vi "Main.vi"(11 "Module Admin":refnum<class "Delacor_lib_QMH_Module Admin.lvclass">) -> ()   [LabVIEW 2019, in "Acquisition.lvlib"]
doc: "This template is based off of the Queued Message Handler design pattern and the Queued Message Handler project template that ships with LabVIEW.\n\nThe main difference is that the queue is private to this module and communication between modules is performed via Broadcast and Request events.\n\nRequest events are wrapped in public API methods and are handled in the Event Handling Loop (EHL) of this VI. Any module can register for Broadcast events sent by this module. The EHL generates messages based on user interface actions.\n\nThe Message Handling Loop (MHL) processes messages generated by the EHL, or by other messages. The messages are string values, so new messages can be added easily to the Message Cases case structure in the MHL. Each message cluster can also provide an optional value for Message Data, which is a variant that can be converted to whatever message-specific data is required.\n_____\nBased on Delacor QMH Project Template 5.0.0.82."
uses:
  Acquisition.lvlib
  <vilib>/Delacor/Delacor QMH/Libraries/Module Admin_class/Delacor_lib_QMH_Module Admin.lvclass
  Module Data--cluster.ctl
  <vilib>/Delacor/Delacor QMH/Libraries/Message Queue_class/Delacor_lib_QMH_Message Queue.lvclass/Delacor_lib_QMH_Message Queue.ctl
  Stop Argument--cluster.ctl
  <vilib>/Delacor/Delacor QMH/Libraries/Module Admin_class/Delacor_lib_QMH_Module Admin.lvclass/Delacor_lib_QMH_Module Admin.ctl
  <vilib>/Utility/miscctls.llb/LVPointTypeDef.ctl
  <vilib>/Delacor/Delacor QMH/Libraries/Message Queue_class/Delacor_lib_QMH_Enqueue Message (Single).vi
  <vilib>/Delacor/Delacor QMH/Libraries/Module Admin_class/Delacor_lib_QMH_Get External Launch.vi
  <vilib>/Utility/error.llb/Error Cluster From Error Code.vi
  <vilib>/ErrorRing/Error Ring.xnode
  <vilib>/Delacor/Delacor QMH/Libraries/Message Queue_class/Delacor_lib_QMH_Message Queue.lvclass
panel:
  in  "Simulate MHL Error":bool
  in  "Simulate EHL Error":bool
  out "error out":errorcluster
  out "Status":string
types:
  T1 = typedef "Acquisition.lvlib/Request Events--cluster.ctl" = cluster{"Stop Module":refnum<user-event>, "Show Panel":refnum<user-event>, "Hide Panel":refnum<user-event>, "Get Module Execution Status":refnum<user-event>, "Show Diagram":refnum<user-event>}
  T2 = typedef "Acquisition.lvlib/Module Data--cluster.ctl" = cluster{"Status":string}
  T3 = enum32{"invalid lock state", "Not Locked", "Locked (No Password)", "Password-protected"}
  T4 = typedef "Acquisition.lvlib/Stop Argument--cluster.ctl" = cluster{"Origin":string, "Exit via Stop Module Req?":bool, "Wait for Module to stop?":bool}
  T5 = typedef "LVPointTypeDef.ctl" = cluster{"Horizontal":i16, "Vertical":i16}
  T6 = enum32{"Invalid", "Standard", "Closed", "Hidden", "Minimized", "Maximized"}
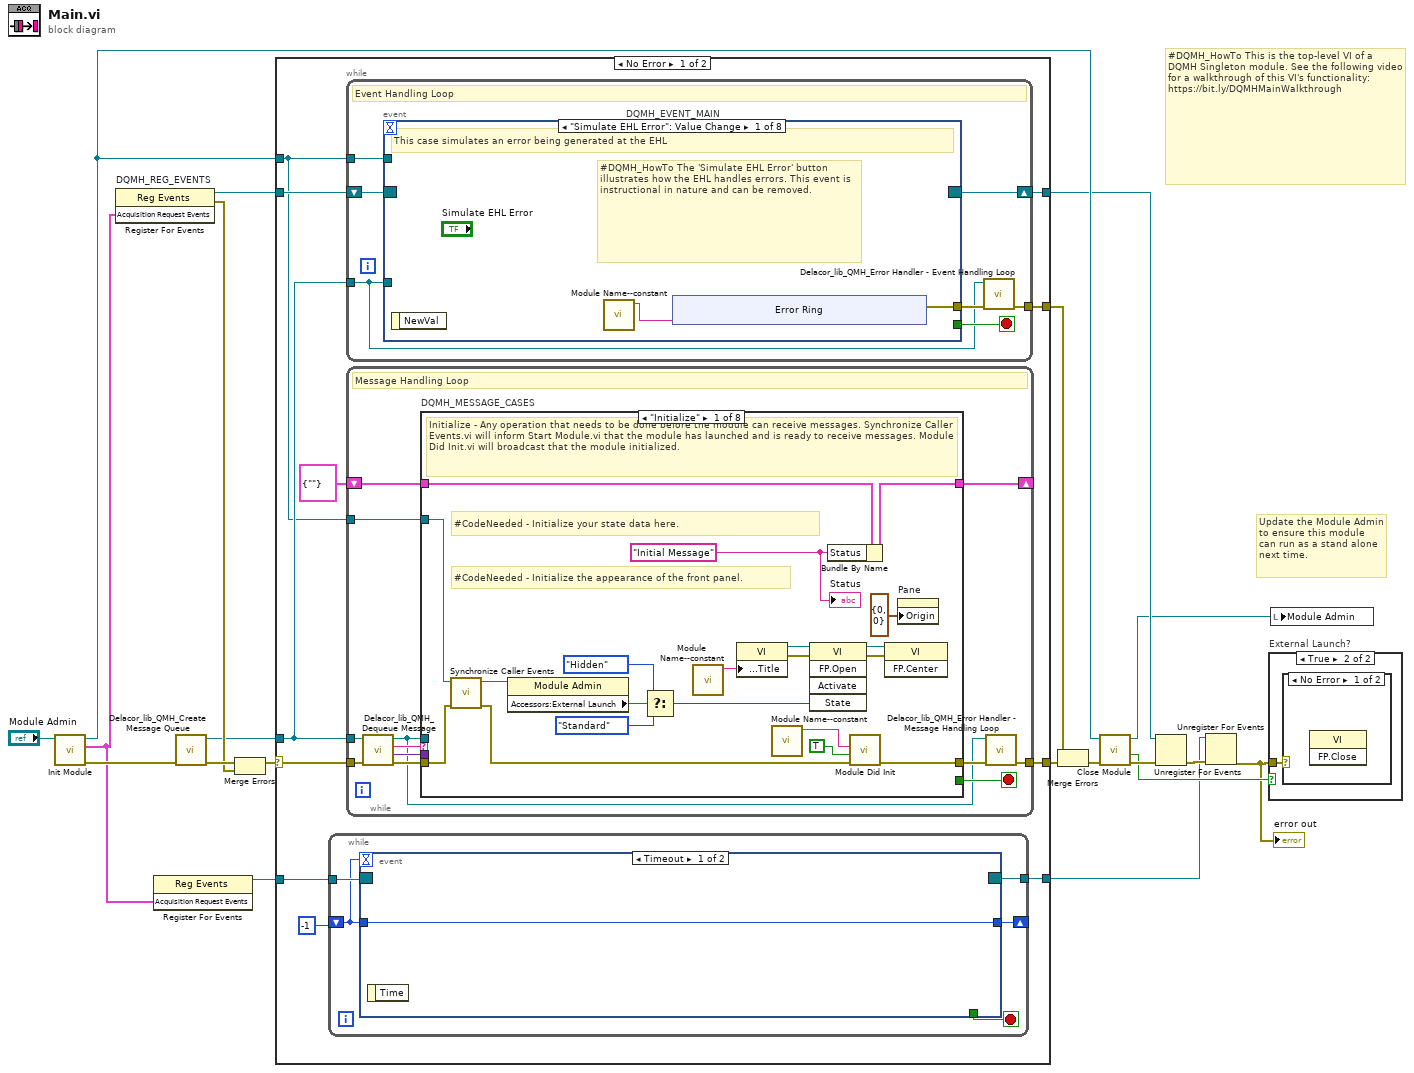
[diagram p0: block diagram]
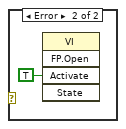
[diagram p3: hidden frame]
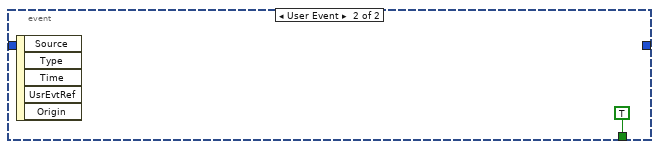
[diagram p4: hidden frame]
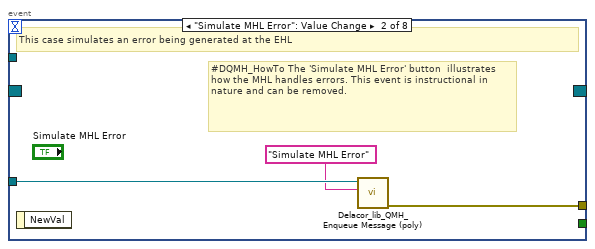
[diagram p5: hidden frame]
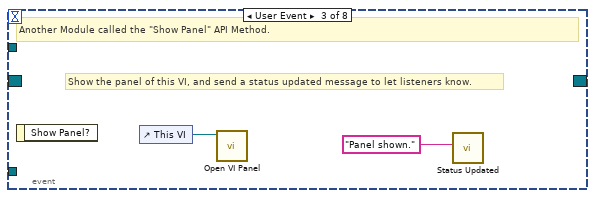
[diagram p6: hidden frame]
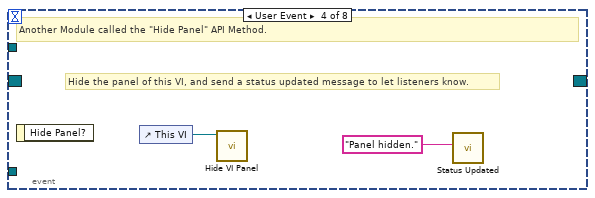
[diagram p7: hidden frame]
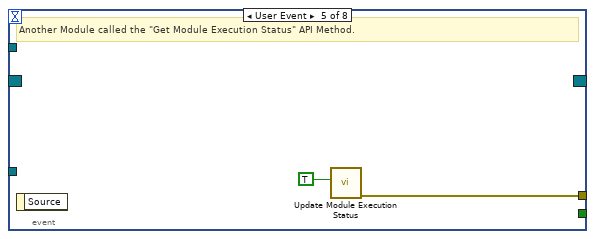
[diagram p8: hidden frame]
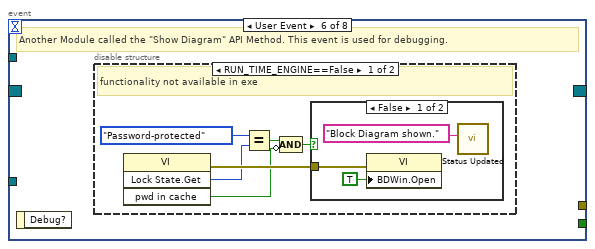
[diagram p9: hidden frame]
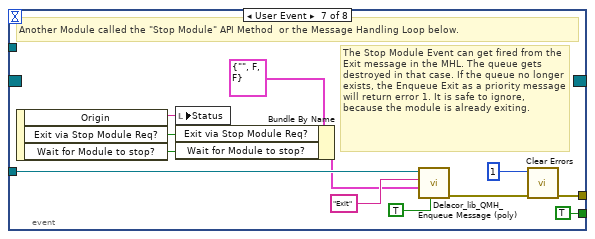
[diagram p12: hidden frame]
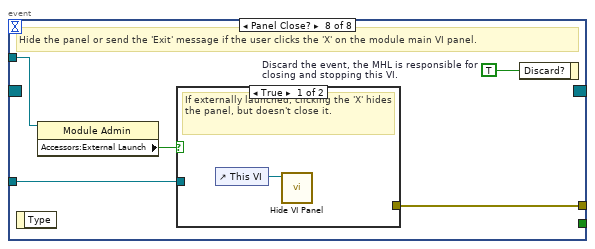
[diagram p13: hidden frame]
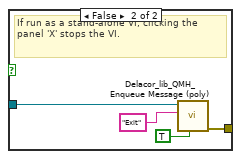
[diagram p14: hidden frame]
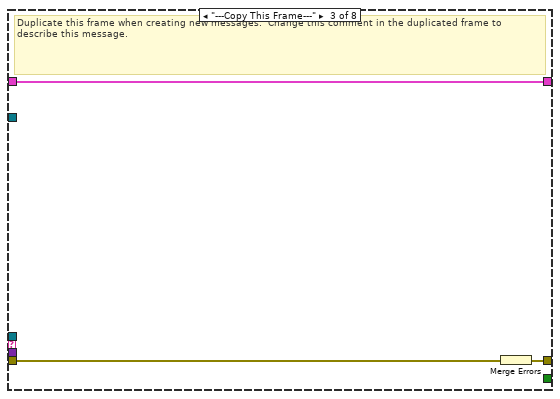
[diagram p16: hidden frame]
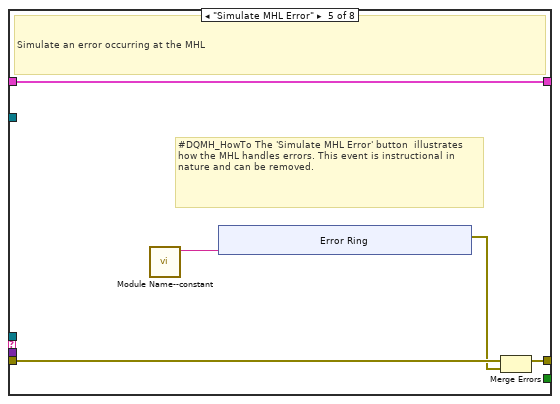
[diagram p18: hidden frame]
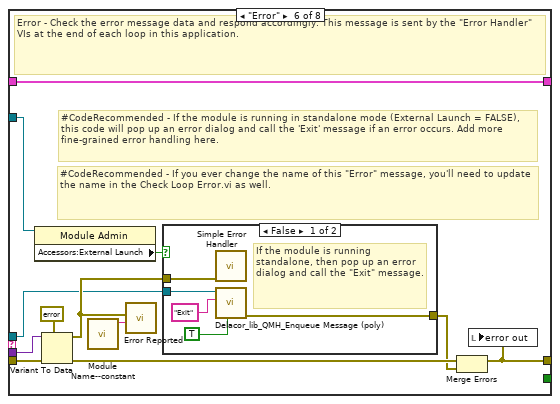
[diagram p19: hidden frame]
diagram:
  # "#DQMH_HowTo This is the top-level VI of a DQMH Singleton module. See the following video for a walkthrough of this VI's functionality: https://bit.ly/DQMHMainWalkthrough"
  # "Update the Module Admin to ensure this module can run as a stand alone next time."
  n1 = call "Init Module.vi"("Singleton Module Admin in"="Module Admin") -> ("error out"=w19:errorcluster, "Acquisition Request Events"=w5:T1, "Singleton Module Admin out"=w12:refnum<class "Delacor_lib_QMH_Module Admin.lvclass">)  [unwired: 8 in]
  n2 = register-events "DQMH_REG_EVENTS"(w5) -> (reference out=w10:refnum<event-registration>, error out=w13:errorcluster)  [unwired: 2 in]
  n3 = register-events(w5) -> (reference out=w4:refnum<event-registration>)  [unwired: 2 in, 1 out]
  n4 = call <vilib>:"Delacor_lib_QMH_Create Message Queue.vi"("error in (no error)"=w19) -> ("error out"=w15:errorcluster, "Message Queue"=w9:refnum<class "Delacor_lib_QMH_Message Queue.lvclass">)  [unwired: 9 in]
  n5 = Merge Errors(w15, w13) -> (w14:errorcluster)
  n6 = case shown="No Error" w14 {
    selector: w14 -> [w29 w195]
    tunnel: [w31 w194] -> w20
    tunnel: [w28 w200] -> w11
    tunnel: w10 -> [w26 w200]
    tunnel: w9 -> [w25 w193]
    tunnel: [w30 _] -> w17
    tunnel: w12 -> [w24 w196]
    tunnel: w4 -> [w23 w192]
    tunnel: [w22 w192] -> w1
    frame No Error {
      n7 = while {
        tunnel: w23 -> [w36]
        tunnel: [w35] -> w22
        shift-right: [w32] -> _
        shift-left: -1 -> [w33]
        stop <- w34 stop-if-true
        n8 = event shown="[0] Timeout" {
          selector: w36 -> [_ _]
          dyn-events: [_ _] -> w35
          timeout: w33 -> [_ _]
          tunnel: [_ TRUE] -> w34
          tunnel: w33 -> [w37 _]
          tunnel: [w37 _] -> w32
          event Timeout {
            n9 = event-data() -> ()  [unwired: 1 in, 1 out]
          }
          event User Event {
            n10 = event-data() -> ()  [unwired: 1 in, 5 out]
          }
        }
      }
      n11 = while {
        tunnel: w25 -> [w39]
        shift-right: [w42] -> w28
        shift-left: w26 -> [w43]
        tunnel: [w44] -> w30
        tunnel: w24 -> [w40]
        stop <- w41 stop-if-true
        # "Event Handling Loop"
        n12 = event "DQMH_EVENT_MAIN" shown="[0] \"Simulate EHL Error\": Value Change" {
          selector: w43 -> [_ _ _ _ _ _ _ _]
          dyn-events: [_ _ _ _ _ _ _ _] -> w42
          timeout: _ -> [_ _ _ _ _ _ _ _]
          tunnel: [_ _ _ _ _ _ TRUE ("Discard?") _] -> w41
          tunnel: w39 -> [_ w56 _ _ _ _ w80 w87]
          tunnel: [w47 w57 _ _ w63 _ w83 w89] -> w45
          tunnel: w40 -> [_ _ _ _ _ _ _ w86]
          event "Simulate EHL Error": Value Change {
            # "#DQMH_HowTo The 'Simulate EHL Error' button  illustrates how the EHL handles errors. This event is instructional in nature and can be removed."
            # "This case simulates an error being generated at the EHL"
            n13 = event-data() -> ()  [unwired: 1 in, 1 out]
            n14 = call "Module Name--constant.vi"() -> ("Module Name"=w46:string)  [unwired: 11 in]
            n15 = xnode "Error Ring"("parameter 0"=w46) -> ("error out"=w47:errorcluster)
          }
          event "Simulate MHL Error": Value Change {
            # "#DQMH_HowTo The 'Simulate MHL Error' button  illustrates how the MHL handles errors. This event is instructional in nature and can be removed."
            # "This case simulates an error being generated at the EHL"
            n16 = event-data() -> ()  [unwired: 1 in, 1 out]
            n17 = call-poly <vilib>:"Delacor_lib_QMH_Enqueue Message (poly).vi"("Message"="Simulate MHL Error", "Message Queue in"=w56) -> ("error out"=w57:errorcluster)  [unwired: 8 in, 1 out]
          }
          event User Event {
            # "Show the panel of this VI, and send a status updated message to let listeners know."
            # "Another Module called the \"Show Panel\" API Method."
            n18 = event-data() -> ()  [unwired: 1 in, 1 out]
            n19 = control-ref of="This VI"() -> (w59:refnum<vi>)
            n20 = call "Open VI Panel.vi"("VI"=w59) -> ()  [unwired: 10 in, 1 out]
            n21 = call "Status Updated.vi"("Status"="Panel shown." ("format string")) -> ()  [unwired: 10 in, 1 out]
          }
          event User Event {
            # "Hide the panel of this VI, and send a status updated message to let listeners know."
            # "Another Module called the \"Hide Panel\" API Method."
            n22 = event-data() -> ()  [unwired: 1 in, 1 out]
            n23 = control-ref of="This VI"() -> (w61:refnum<vi>)
            n24 = call "Hide VI Panel.vi"("VI"=w61) -> ()  [unwired: 10 in, 1 out]
            n25 = call "Status Updated.vi"("Status"="Panel hidden." ("format string")) -> ()  [unwired: 10 in, 1 out]
          }
          event User Event {
            # "Another Module called the \"Get Module Execution Status\" API Method."
            n26 = event-data() -> ()  [unwired: 1 in, 1 out]
            n27 = call "Update Module Execution Status.vi"("Running?"=TRUE) -> ("error out"=w63:errorcluster)  [unwired: 10 in]
          }
          event User Event {
            # "Another Module called the \"Show Diagram\" API Method. This event is used for debugging."
            n28 = event-data() -> ()  [unwired: 1 in, 1 out]
            n29 = disable-structure shown="RUN_TIME_ENGINE==False" {
              frame condition #0 (active) {
                # "functionality not available in exe"
                n30 = invoke class="VI" method="Lock State.Get"() -> (error out=w69:errorcluster, "Get Lock State"=w68:T3, "pwd in cache"=w65:bool)  [unwired: 4 in, 1 out]
                n31 = Equal?(x=T3."Password-protected", y=w68) -> (x = y?=w66:bool)
                n32 = Compound Arithmetic op=AND(w66, invert w65) -> (w64:bool)
                n33 = case shown="False" w64 {
                  tunnel: w69 -> [w72 _]
                  frame False {
                    n34 = property class="VI"(error in=w72, "BDWin.Open"=TRUE ("Block Diagram Window:Open")) -> ()  [unwired: 1 in, 2 out]
                    n35 = call "Status Updated.vi"("Status"="Block Diagram shown." ("format string")) -> ()  [unwired: 10 in, 1 out]
                  }
                  frame True {
                    # "Password-protected VI, and the password is not in the cache. Do not show the diagram."
                  }
                }
              }
              frame condition #1 {
              }
            }
          }
          event User Event {
            # "The Stop Module Event can get fired from the Exit message in the MHL. The queue gets destroyed in that case. If the queue no longer exists, the Enqueue Exit as a priority message will return error 1. It is safe to ignore, because the module is already exiting."
            # "Another Module called the \"Stop Module\" API Method  or the Message Handling Loop below."
            n36 = event-data() -> ("Origin"=w79:string, "Exit via Stop Module Req?"=w75:bool, "Wait for Module to stop?"=w74:bool)  [unwired: 1 in]
            n37 = local write "Status"(w79) -> ()
            n38 = Bundle By Name(cluster=T4 {"Origin"="", "Exit via Stop Module Req?"=FALSE, "Wait for Module to stop?"=FALSE} ("Stop Argument"), "Exit via Stop Module Req?"=w75, "Wait for Module to stop?"=w74) -> (w73:T4)
            n39 = call-poly <vilib>:"Delacor_lib_QMH_Enqueue Message (poly).vi"("Priority Message? (F)"=TRUE, "Message Data"=w73, "Message"="Exit", "Message Queue in"=w80) -> ("error out"=w84:errorcluster)  [unwired: 6 in, 1 out]
            n40 = call <vilib>:"Clear Errors.vi"("error in (no error)"=w84, "specific error code to clear (0: all)"=1) -> ("error out"=w83:errorcluster)  [unwired: 4 in, 1 out]
          }
          event Panel Close? {
            w88 = TRUE  # Discard the event, the MHL is responsible for closing and stopping this VI.
            # "Hide the panel or send the 'Exit' message if the user clicks the 'X' on the module main VI panel."
            n41 = event-data() -> ()  [unwired: 1 in, 1 out]
            n42 = property class="Module Admin"(reference=w86) -> ("Accessors:External Launch"=w85:bool)  [unwired: 1 in, 2 out]
            n43 = case shown="True" w85 {
              tunnel: w87 -> [_ w93]
              tunnel: [_ w94] -> w89
              frame True {
                # "If externally launched, clicking the 'X' hides the panel, but doesn't close it."
                n44 = control-ref of="This VI"() -> (w90:refnum<vi>)
                n45 = call "Hide VI Panel.vi"("VI"=w90) -> ()  [unwired: 10 in, 1 out]
              }
              frame False {
                # "If run as a stand-alone VI, clicking the panel 'X' stops the VI."
                n46 = call-poly <vilib>:"Delacor_lib_QMH_Enqueue Message (poly).vi"("Priority Message? (F)"=TRUE, "Message"="Exit", "Message Queue in"=w93) -> ("error out"=w94:errorcluster)  [unwired: 7 in, 1 out]
              }
            }
            n47 = event-data("Discard?"=w88) -> ()  [unwired: 1 in, 1 out]
          }
        }
        n48 = call-dynamic "Delacor_lib_QMH_Error Handler - Event Handling Loop.vi"("error in (no error)"=w45, "Message Queue in"=w39) -> ("dup error in"=w44:errorcluster)  [unwired: 8 in, 1 out]
      }
      n49 = while {
        tunnel: w25 -> [w97]
        shift-right: [w101] -> _
        shift-left: T2 {"Status"=""} ("Data Cluster") -> [w102]
        tunnel: w29 -> [w105]
        tunnel: [w103] -> w31
        tunnel: w24 -> [w95]
        stop <- w100 stop-if-true
        # "Message Handling Loop"
        n50 = call-dynamic "Delacor_lib_QMH_Dequeue Message.vi"("error in (no error)"=w105, "Message Queue in"=w97) -> ("error out"=w104:errorcluster, "Message Data"=w98:variant, "Message"=w99:string, "Message Queue out"=w96:refnum<class "Delacor_lib_QMH_Message Queue.lvclass">)  [unwired: 6 in]
        n51 = case "DQMH_MESSAGE_CASES" shown="\"Initialize\"" w99 {
          selector: w99 -> [_ _ _ _ _ _ _ w179]
          tunnel: w96 -> [_ _ _ _ _ w149 w171 _]
          tunnel: w104 -> [w124 w128 w131 w133 w138 w156 w177 w181]
          tunnel: [w122 w128 w130 w133 w137 w152 w174 w182] -> w106
          tunnel: w102 -> [w113 w127 w129 w132 w135 w151 w170 w180]
          tunnel: [w112 w127 w129 w132 w135 w151 w170 w180] -> w101
          tunnel: [_ _ _ _ _ _ w169 _] -> w100
          tunnel: w98 -> [_ _ _ _ _ w150 w168 _]
          tunnel: w95 -> [w114 _ _ _ _ w148 w163 _]
          frame "Initialize" {
            w107 = "Initial Message" ("Initial Message")
            # "#CodeNeeded - Initialize the appearance of the front panel."
            # "#CodeNeeded - Initialize your state data here."
            # "Initialize - Any operation that needs to be done before the module can receive messages. Synchronize Caller Events.vi will inform Start Module.vi that the module has launched and is ready to receive messages. Module Did Init.vi will broadcast that the module initialized."
            n52 = call "Synchronize Caller Events.vi"("error in (no error)"=w124, "Singleton Module Admin in"=w114) -> ("error out"=w123:errorcluster, "Singleton Module Admin out"=w109:refnum<class "Delacor_lib_QMH_Module Admin.lvclass">)  [unwired: 8 in]
            n53 = property class="Module Admin"(reference=w109) -> ("Accessors:External Launch"=w118:bool)  [unwired: 1 in, 2 out]
            n54 = Select(t=T6."Hidden" ("State"), s=w118, f=T6."Standard" ("State")) -> (s? t:f=w115:T6)
            n55 = call "Module Name--constant.vi"() -> ("Module Name"=w121:string)  [unwired: 11 in]
            n56 = property class="VI"("Front Panel.Title"=w121) -> (reference out=w120:refnum<vi>, error out=w126:errorcluster)  [unwired: 2 in]
            n57 = call "Module Name--constant.vi"() -> ("Module Name"=w110:string)  [unwired: 11 in]
            n58 = invoke class="VI" method="FP.Open"(reference=w120, error in=w126, "State"=w115) -> (reference out=w119:refnum<vi>, error out=w125:errorcluster)  [unwired: 2 in, 3 out]
            n59 = Bundle By Name(cluster=w113, "Status"=w107) -> (w112:T2)
            n60 = call "Module Did Init.vi"("error in (no error)"=w123, "Initialized?"=TRUE, "Origin"=w110) -> ("error out"=w122:errorcluster)  [unwired: 8 in]
            n61 = invoke class="VI" method="FP.Center"(reference=w119, error in=w125) -> ()  [unwired: 1 in, 3 out]
            n62 = property on="Pane" class="Pane"("Origin"=T5 {"Horizontal"=0, "Vertical"=0}) -> ()  [unwired: 2 in, 2 out]
            "Status" <- w107
          }
          frame "--- Module Specific ---" {
            # "Separator -- The following cases handle messages specific to this Module."
          }
          frame "---Copy This Frame---" {
            # "Duplicate this frame when creating new messages.  Change this comment in the duplicated frame to describe this message."
            n63 = Merge Errors(w131) -> (w130:errorcluster)
          }
          frame "--- Exit and Error Handling---" {
            # "Separator - The following cases handle errors and exit messages."
          }
          frame "Simulate MHL Error" {
            # "#DQMH_HowTo The 'Simulate MHL Error' button  illustrates how the MHL handles errors. This event is instructional in nature and can be removed."
            # "Simulate an error occurring at the MHL"
            n64 = call "Module Name--constant.vi"() -> ("Module Name"=w134:string)  [unwired: 11 in]
            n65 = xnode "Error Ring"("parameter 0"=w134) -> ("error out"=w136:errorcluster)
            n66 = Merge Errors(w138, w136) -> (w137:errorcluster)
          }
          frame "Error" {
            # "#CodeRecommended - If you ever change the name of this \"Error\" message, you'll need to update the name in the Check Loop Error.vi as well."
            # "#CodeRecommended - If the module is running in standalone mode (External Launch = FALSE), this code will pop up an error dialog and call the 'Exit' message if an error occurs. Add more fine-grained error handling here."
            # "Error - Check the error message data and respond accordingly. This message is sent by the \"Error Handler\" VIs at the end of each loop in this application."
            n67 = property class="Module Admin"(reference=w148) -> ("Accessors:External Launch"=w147:bool)  [unwired: 1 in, 2 out]
            n68 = Variant To Data(error in=w156, type=errorcluster {"status"=FALSE, "code"=0, "source"=""} ("error constant"), Variant=w150) -> (data=w157:errorcluster, error out=w154:errorcluster)
            n69 = call "Module Name--constant.vi"() -> ("Module Name"=w146:string)  [unwired: 11 in]
            n70 = call "Error Reported.vi"("Additional Information"=w146, "Error"=w157) -> ()  [unwired: 9 in, 1 out]
            n71 = case shown="False" w147 {
              tunnel: [w162 _] -> w153
              tunnel: w149 -> [w160 _]
              tunnel: w157 -> [w161 _]
              frame False {
                # "If the module is running standalone, then pop up an error dialog and call the \"Exit\" message."
                n72 = call <vilib>:"Simple Error Handler.vi"("error in (no error)"=w161) -> ()  [unwired: 4 in, 5 out]
                n73 = call-poly <vilib>:"Delacor_lib_QMH_Enqueue Message (poly).vi"("Priority Message? (F)"=TRUE, "Message"="Exit", "Message Queue in"=w160) -> ("error out"=w162:errorcluster)  [unwired: 7 in, 1 out]
              }
              frame True {
                # "If the module was launched externally, calling the Error Reported broadcast VI is the only action performed by the \"Error\" message. The module's caller can then process the error appropriately."
              }
            }
            n74 = Merge Errors(w154, w153) -> (w152:errorcluster)
            n75 = local write "error out"(w152) -> ()
          }
          frame "Exit" {
            w167 = 91  # 91: not all Exit messages will have an argument
            w169 = TRUE  # Stop the VI
            # "Release the message queue reference"
            # "#CodeNeeded - Add any required cleanup code here"
            # "Exit - Exit the application."
            n76 = Variant To Data(error in=w177, type=T4 {"Origin"="", "Exit via Stop Module Req?"=FALSE, "Wait for Module to stop?"=FALSE} ("Stop Argument"), Variant=w168) -> (data=w165:T4, error out=w173:errorcluster)
            n77 = call <vilib>:"Clear Errors.vi"("error in (no error)"=w173, "specific error code to clear (0: all)"=w167) -> ("error out"=w176:errorcluster)  [unwired: 4 in, 1 out]
            n78 = control-ref of="This VI"() -> (w164:refnum<vi>)
            n79 = call-dynamic "Delacor_lib_QMH_Release Message Queue.vi"("error in (no error)"=w176, "Message Queue"=w171) -> ("error out"=w175:errorcluster)  [unwired: 9 in]
            n80 = call "Handle Exit.vi"("Stop Argument"=w165, "Admin in"=w163, "VI reference"=w164) -> ("error out"=w172:errorcluster)  [unwired: 7 in, 1 out]
            n81 = Merge Errors(w175, w172) -> (w174:errorcluster)
          }
          frame Default {
            # "'Default' case only runs if there is a message that isn't defined in any of the other cases.  Output a programming error."
            n82 = call "Module Name--constant.vi"() -> ("Module Name"=w178:string)  [unwired: 11 in]
            n83 = xnode "Error Ring"("parameter 0"=w179, "parameter 1"=w178) -> ("error out"=w183:errorcluster)
            n84 = Merge Errors(w181, w183) -> (w182:errorcluster)
          }
        }
        n85 = call-dynamic "Delacor_lib_QMH_Error Handler - Message Handling Loop.vi"("error in (no error)"=w106, "Message Queue in"=w96) -> ("dup error in"=w103:errorcluster)  [unwired: 8 in, 1 out]
      }
    }
    frame Error {
      # "Synchronize Caller Events.vi will inform Start Module.vi that the module has launched and will let the code calling Start Module.vi register for broadcasts and would permit the caller receive the broadcast that an error occurred at launch time."
      n86 = call-dynamic "Delacor_lib_QMH_Release Message Queue.vi"("error in (no error)"=w195, "Message Queue"=w193) -> ("error out"=w194:errorcluster)  [unwired: 9 in]
      n87 = call "Synchronize Caller Events.vi"("Singleton Module Admin in"=w196) -> ("error out"=w201:errorcluster)  [unwired: 9 in, 1 out]
      n88 = call "Module Name--constant.vi"() -> ("Module Name"=w199:string)  [unwired: 11 in]
      n89 = Format Into String(format string="An error occurred during initialization. %s is no longer running.", w199) -> (resulting string=w197:string)  [unwired: 2 in, 1 out]
      n90 = Merge Errors(w194, w201) -> (w202:errorcluster)
      n91 = call "Error Reported.vi"("Additional Information"=w197, "Error"=w202) -> ()  [unwired: 9 in, 1 out]
    }
  }
  n92 = Merge Errors(w17, w20) -> (w16:errorcluster)
  n93 = call "Close Module.vi"("error in (no error)"=w16, "Module Admin in"=w12) -> ("error out"=w18:errorcluster, "External Launch"=w6:bool, "Module Admin out"=w7:refnum<class "Delacor_lib_QMH_Module Admin.lvclass">)  [unwired: 7 in]
  n94 = Unregister For Events(event registration refnum=w11, error in=w18) -> (error out=w3:errorcluster)
  n95 = Unregister For Events(event registration refnum=w1, error in=w3) -> (error out=w2:errorcluster)
  "error out" <- w2
  n96 = case "External Launch?" shown="True" w6 {
    tunnel: w2 -> [_ w203]
    frame False {
    }
    frame True {
      n97 = case shown="No Error" w203 {
        frame No Error {
          n98 = invoke class="VI" method="FP.Close"() -> ()  [unwired: 3 in, 3 out]
        }
        frame Error {
          n99 = invoke class="VI" method="FP.Open"("Activate"=TRUE ("Activate?")) -> ()  [unwired: 4 in, 5 out]
        }
      }
    }
  }
  n100 = local write "Module Admin"(w7) -> ()
